vi "Parse-attribute.vi"(8 "error in (no error)":errorcluster, 10 "String in":string, 11 "JumpSpeed in":refnum<class "JumpSpeed.lvclass">) -> (0 "error out":errorcluster, 1 "Valid attribute?":bool, 2 "Remaining string":string, 3 "JumpSpeed out":refnum<class "JumpSpeed.lvclass">)   [LabVIEW 2013, in "MaterialCharacterization.lvlib" / "JumpSpeed.lvclass"]
uses:
  JumpSpeed.lvclass
  Attributes.ctl
  Attribute-ID.ctl
  Attribute-XML.lvclass/Attribute-XML.ctl
  ID.lvclass/ID.ctl
  Speed/Speed.lvclass/Speed.ctl
  Write Attribute.vi
  Write ID-attribute.vi
  Speed/Write Speed.vi
  Speed/Write Update period.vi
  Speed/Write Bits per period.vi
  Speed/Write Components.vi
  Attribute-XML.lvclass
  ID.lvclass
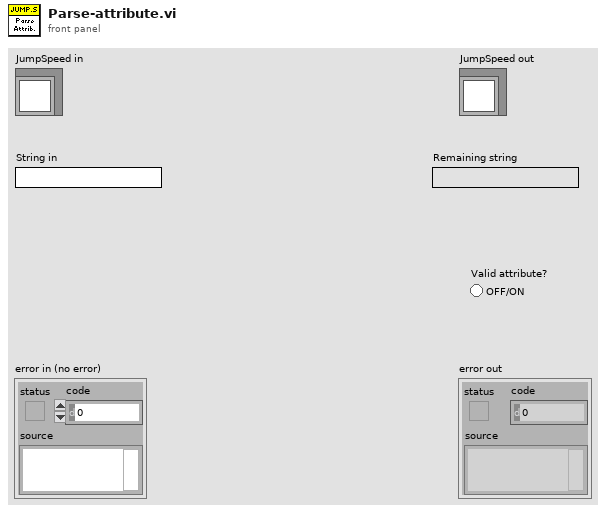
[diagram p1: front panel]
types:
  T1 = typedef "MaterialCharacterization.lvlib/ID.lvclass/Attribute-ID.ctl" = enum16{"FieldOffset", "TransformEnable", "Transform", "Units", "XYCalFactor", "EnableLaser", "JumpDelay", "MarkDelay", "PolyDelay", "LaserOnDelay", "LaserOffDelay", "JumpSpeed", "MarkSpeed", "LaserPowerDelay", "LaserEnableDelay", "LaserPower", "Offset"}
  T2 = typedef "MaterialCharacterization.lvlib/Attribute-XML.lvclass/Attributes.ctl" = enum16{"id"}
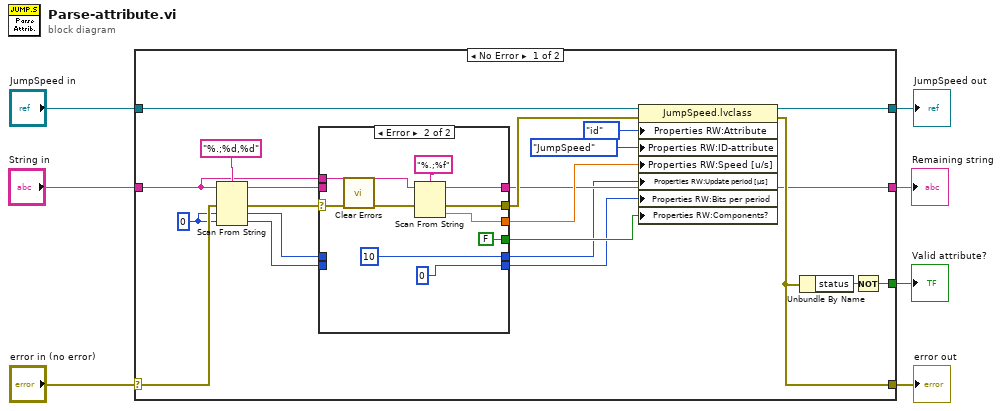
[diagram p0: block diagram]
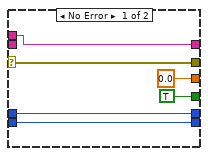
[diagram p2: hidden frame]
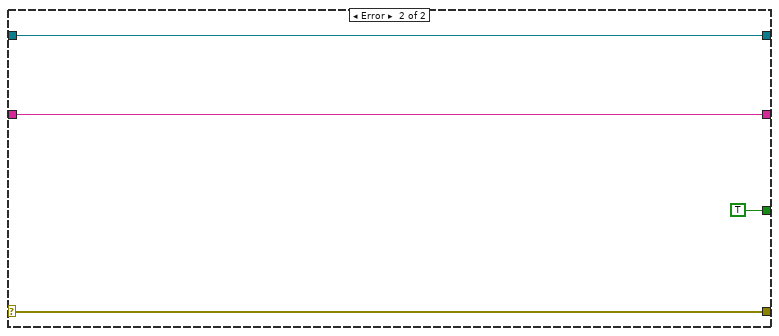
[diagram p3: hidden frame]
diagram:
  n1 = case shown="No Error" "error in (no error)" {
    selector: "error in (no error)" -> [w21 w48]
    tunnel: [w20 w48] -> w6
    tunnel: [w23 w47] -> w4
    tunnel: "JumpSpeed in" -> [w24 w47]
    tunnel: "String in" -> [w15 w46]
    tunnel: [w10 w46] -> w2
    tunnel: [w22 TRUE] -> w1
    frame No Error {
      w19 = u16 0 ("default value 2")
      n2 = Scan From String(format string="%.;%d,%d", input string=w15, error in=w21, default 1=w19, default 2=w19) -> (remaining string=w14:string, error out=w18:errorcluster, output 1=w17:u16, output 2=w16:u16)  [unwired: 1 in, 1 out]
      n3 = case shown="Error" w18 {
        selector: w18 -> [w30 w43]
        tunnel: w17 -> [w34 _]
        tunnel: w16 -> [w33 _]
        tunnel: w15 -> [w29 w42]
        tunnel: w14 -> [_ _]
        tunnel: [w30 w41] -> w13
        tunnel: [0.0 w40] -> w12
        tunnel: [TRUE FALSE] -> w11
        tunnel: [w29 w38] -> w10
        tunnel: [w34 u16 10 ("default value 2")] -> w9
        tunnel: [w33 u16 0 ("default value 2")] -> w8
        frame No Error {
        }
        frame Error {
          n4 = call <vilib>:"Clear Errors.vi"("error in (no error)"=w43) -> ("error out"=w37:errorcluster)  [unwired: 6 in]
          n5 = Scan From String(format string="%.;%f", input string=w42, error in=w37) -> (remaining string=w38:string, error out=w41:errorcluster, output 1=w40:dbl)  [unwired: 2 in, 1 out]
        }
      }
      n6 = property class="JumpSpeed.lvclass"(reference=w24, error in=w13, "Properties RW:Attribute"=Attributes."id" ("Attribute"), "Properties RW:ID-attribute"=Attribute-ID."JumpSpeed" ("ID-attribute"), "Properties RW:Speed [u/s]"=w12, "Properties RW:Update period [µs]"=w9, "Properties RW:Bits per period"=w8, "Properties RW:Components?"=w11) -> (reference out=w23:refnum<class "JumpSpeed.lvclass">, error out=w20:errorcluster)
      n7 = Unbundle By Name(w20) -> ("status"=w27:bool)
      n8 = Not(x=w27) -> (.not. x?=w22:bool)
    }
    frame Error {
    }
  }
  "error out" <- w6
  "JumpSpeed out" <- w4
  "Remaining string" <- w2
  "Valid attribute?" <- w1
